vi "Get AI Ranges.vi"(0 "Module Ref":refnum<class "Modbus Master.lvclass">, 11 "error in (no error)":errorcluster) -> (4 "Modbus master out":refnum<class "Modbus Master.lvclass">, 6 "Channel Ranges":T1[](array[typedef]) items=["+-150mV", "+-500mV", "0~150mV", "0~500mV", "+-1V", "+-5V", "+-10V", "0~1V", "0~5V", "0~10V", "+-20mA", "4~20mA", "0~20mA"], 15 "error out":errorcluster)   [LabVIEW 2024]
doc: "Read back analogue input measurment ranges."
uses:
  <vilib>/NI/Modbus Library/API/Master/Modbus Master.lvclass
  Support VIs/Range.ctl
panel:
  # "Channel 0"
  # "Channel 1"
  # "Channel 2"
  # "Channel 3"
  # "Channel 4"
  # "Channel 5"
  # "Channel 6"
  # "Channel 7"
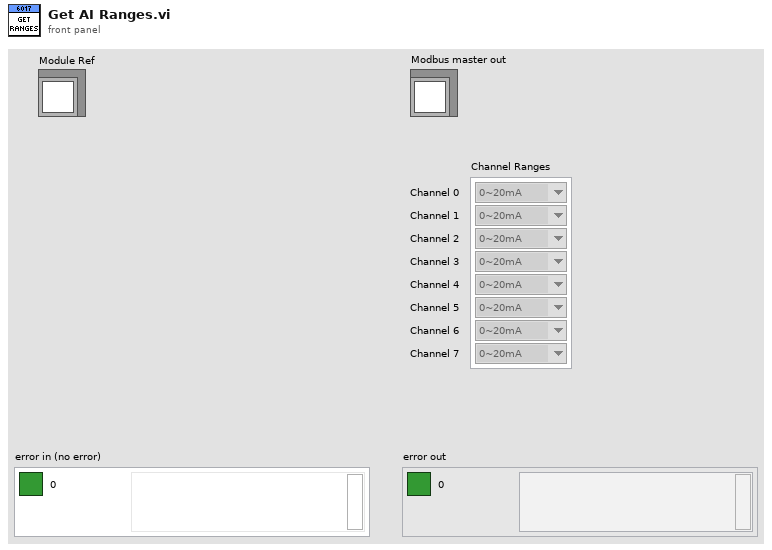
[diagram p1: front panel]
types:
  T1 = typedef "Range.ctl" = u16
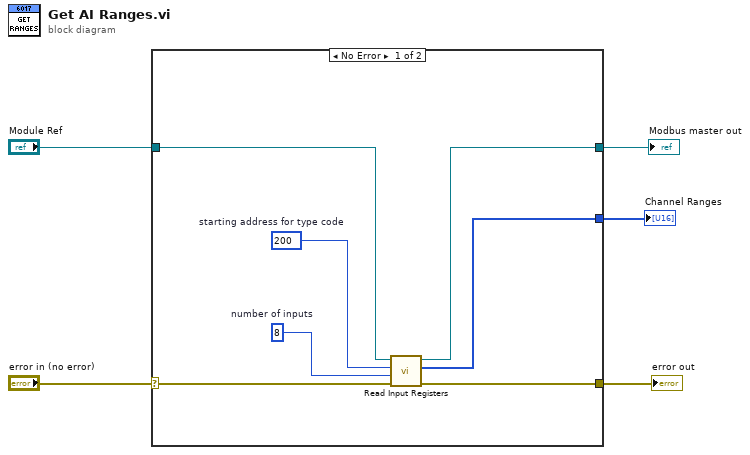
[diagram p0: block diagram]
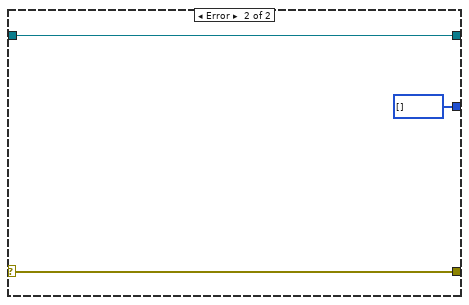
[diagram p2: hidden frame]
diagram:
  n1 = case shown="No Error" "error in (no error)" {
    selector: "error in (no error)" -> [w12 w14]
    tunnel: "Module Ref" -> [w11 w15]
    tunnel: [w8 w15] -> w3
    tunnel: [w7 w14] -> w2
    tunnel: [w6 u16[] [] ("register values")] -> w1
    frame No Error {
      w9 = u16 200  # starting address for type code
      w10 = u16 8  # number of inputs
      n2 = call-dynamic "Read Input Registers.vi"("error in"=w12, "number of inputs"=w10, "starting address"=w9, "Modbus master in"=w11) -> ("error out"=w7:errorcluster, "register values"=w6:u16[], "Modbus master out"=w8:refnum<class "Modbus Master.lvclass">)  [unwired: 5 in]
    }
    frame Error {
    }
  }
  "error out" <- w2
  "Modbus master out" <- w3
  "Channel Ranges" <- w1
